vi "Sample Main.vi"() -> ()   [LabVIEW 2023]
doc: "This is a sample main VI that will be built into an executable."
panel:
  in  "Stop":bool
  out "Waveform Chart":dbl(graph)
  # "This is a sample main VI that will be built into an executable."
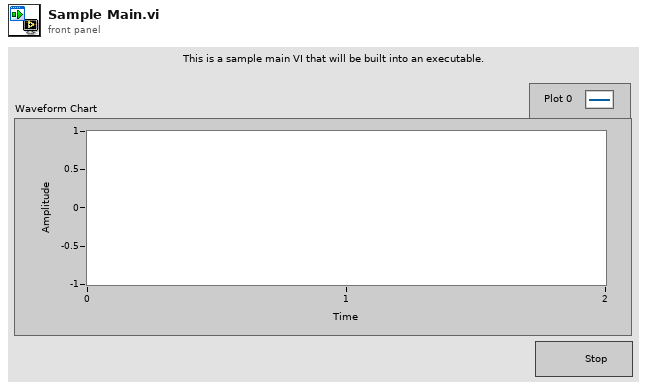
[diagram p1: front panel]
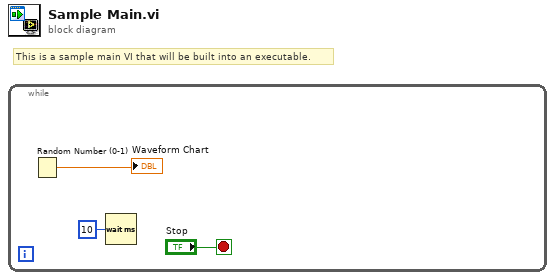
[diagram p0: block diagram]
diagram:
  # "This is a sample main VI that will be built into an executable."
  n1 = while {
    stop <- "Stop" stop-if-true
    n2 = Random Number (0-1)() -> (number: 0 to 1=→"Waveform Chart":dbl)
    n3 = Wait (ms)(milliseconds to wait=u32 10) -> ()  [unwired: 1 out]
  }
